vi "ini_file.vi"(0 "device_type in":refnum<class "device_type.lvclass">, 11 "error in (no error)":errorcluster) -> (4 "device_type out":refnum<class "device_type.lvclass">, 6 "Numeric":i32, 15 "error out":errorcluster)   [LabVIEW 2021, in "device_type.lvclass"]
uses:
  device_type.lvclass
  device_type.lvclass/device_type.ctl
panel:
  out "Numeric 2":i32
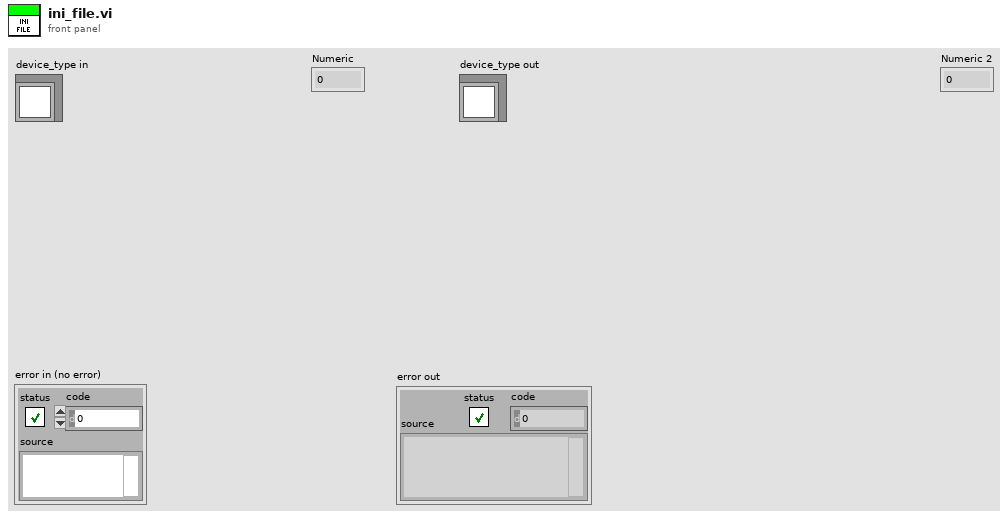
[diagram p1: front panel]
types:
  T1 = enum16{"open", "open or create", "create or replace", "create", "open (read-only)"}
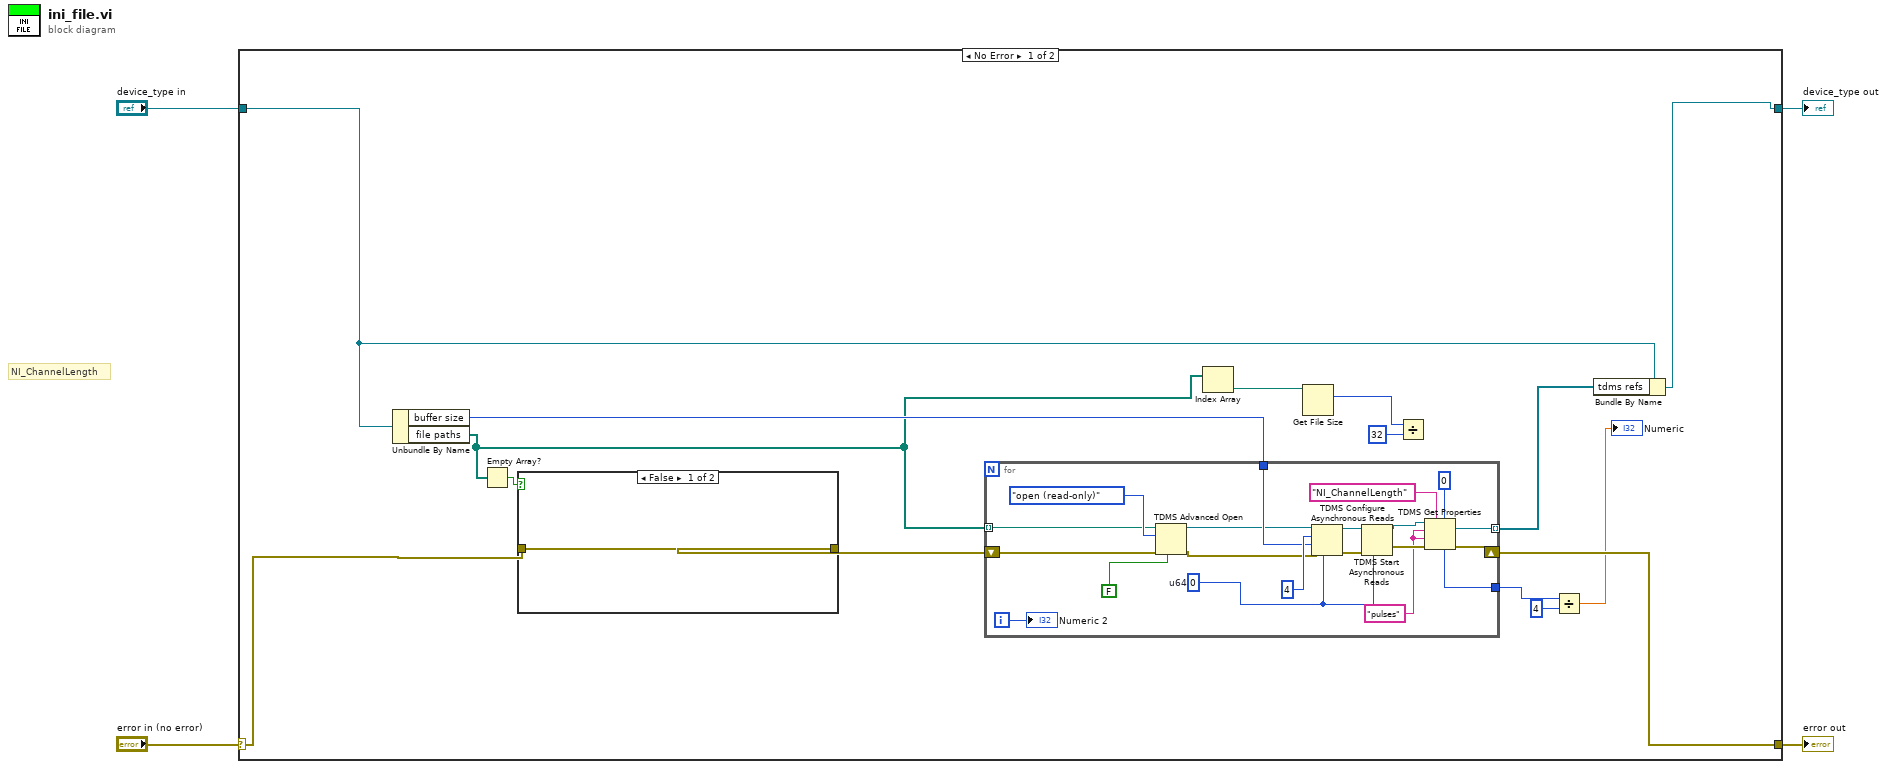
[diagram p0: block diagram]
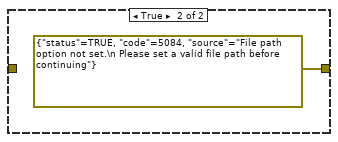
[diagram p2: hidden frame]
diagram:
  # "NI_ChannelLength"
  n1 = case shown="No Error" "error in (no error)" {
    selector: "error in (no error)" -> [w8 w43]
    tunnel: [w9 w43] -> w3
    tunnel: [w10 w42] -> w1
    tunnel: "device_type in" -> [w11 w42]
    frame No Error {
      n2 = Unbundle By Name(w11) -> ("buffer size"=w19:u32, "file paths"=w13:path[])
      n3 = Empty Array?(array=w13) -> (empty?=w14:bool)
      n4 = case shown="False" w14 {
        tunnel: [w20 errorcluster {"status"=TRUE, "code"=5084, "source"="File path option not set.\n Please set a valid file path before continuing"} ("error in (no error)")] -> w12
        tunnel: w8 -> [w20 _]
        frame False {
        }
        frame True {
        }
      }
      n5 = for {
        tunnel: w13 -> [w31] mode=indexing
        tunnel: [w26] -> w18 mode=indexing
        shift-right: [w27] -> w9
        shift-left: w12 -> [w36]
        tunnel: w19 -> [w34]
        tunnel: [w23] -> w7
        i -> [w30]
        w22 = "pulses" ("channel name")
        w35 = u64 0  # u64
        n6 = TDMS Advanced Open(6:FALSE ("Disable Buffering? (T)"), 8:w36, 10:T1."open (read-only)" ("Operation"), 11:w31) -> (0:w37:errorcluster, 3:w33:refnum<k34>)  [unwired: 1 in, 1 out]
        n7 = TDMS Configure Asynchronous Reads(6:w35, 8:w37, 9:w34, 10:u32 4 ("Number of Buffers (4)"), 11:w33) -> (0:w39:errorcluster, 3:w32:refnum<k34>)  [unwired: 1 in]
        n8 = TDMS Start Asynchronous Reads(6:w35, 8:w39, 11:w32) -> (0:w28:errorcluster, 3:w29:refnum<k34>)  [unwired: 1 in]
        n9 = TDMS Get Properties(5:u64 0, 7:"NI_ChannelLength" ("property name"), 8:w28, 9:w22, 10:w22, 11:w29) -> (0:w27:errorcluster, 3:w26:refnum<k34>, 4:w23:u64)  [unwired: 3 out]
        "Numeric 2" <- w30
      }
      n10 = Index Array(array=w13) -> (element=w17:path)  [unwired: 1 in]
      n11 = Get File Size(file=w17) -> (size (in bytes)=w16:i64)  [unwired: 1 in, 2 out]
      n12 = Divide(x=w16, y=i64 32) -> ()  [unwired: 1 out]
      n13 = Divide(x=w7, y=u64 4) -> (x/y=→"Numeric":dbl)
      n14 = Bundle By Name(cluster=w11, "tdms refs"=w18) -> (w10:refnum<class "device_type.lvclass">)
    }
    frame Error {
    }
  }
  "error out" <- w3
  "device_type out" <- w1
